vi "Build Address Tree.vi"(8 "error in (no error)":errorcluster, 10 "variant":variant, 11 "Addresses":refnum<vi>) -> (0 "error out":errorcluster, 2 "duplicate variant":variant)   [LabVIEW 2019, in "J1939 Workspace Shared.lvlib"]
uses:
  J1939 Workspace Shared.lvlib
  <vilib>/Utility/miscctls.llb/LVNodeAndColumnTypeDef.ctl
  <vilib>/picture/picture.llb/imagedata.ctl
  Addon/Addon Shared/Types/Address Lookup Table Data.ctl
  Addon/Addon Shared/J1939 Addon Shared.lvlib
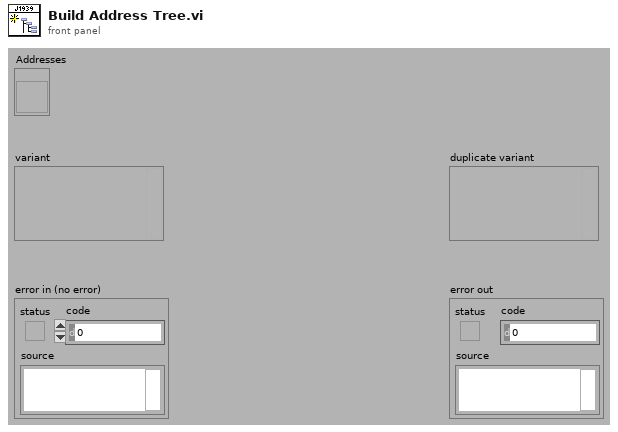
[diagram p1: front panel]
types:
  T1 = typedef "LVNodeAndColumnTypeDef.ctl" = cluster{"Node":string, "Column":i32}
  T2 = typedef "imagedata.ctl" = cluster{"image type":i32, "image depth":i32, "image":u8[], "mask":u8[], "colors":u32[], "Rectangle":cluster{"left":i16, "top":i16, "right":i16, "bottom":i16}}
  T3 = typedef "J1939 Addon Shared.lvlib/Address Lookup Table Data.ctl" = cluster{"Name":u8[], "Address":u8}
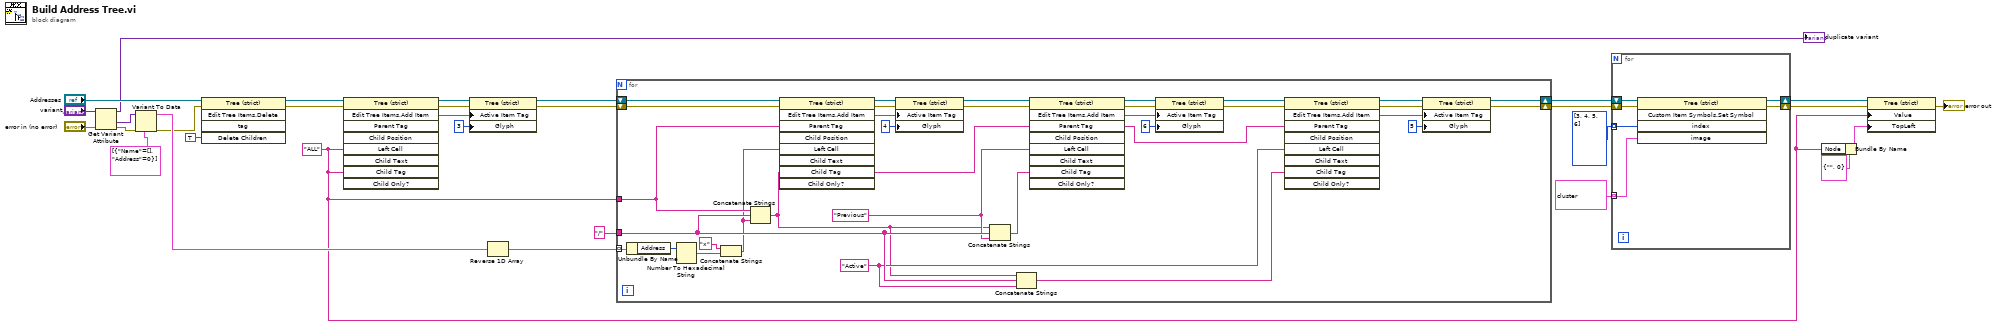
[diagram p0: block diagram]
diagram:
  w3 = "ALL" ("Left Cell String")
  n1 = Get Variant Attribute(Variant="variant", error in="error in (no error)") -> (duplicate Variant=→"duplicate variant":variant, values=w22:variant[], error out=w23:errorcluster)  [unwired: 2 in, 1 out]
  n2 = Variant To Data(error in=w23, type=T3[] [{"Name"=[], "Address"=0}], Variant=w22) -> (data=w21:T3[], error out=w18:errorcluster)
  n3 = invoke on="Invoke Node" class="Tree (strict)" method="Edit Tree Items.Delete"(reference="Addresses", error in=w18, "Delete Children"=TRUE ("Delete Children?")) -> (reference out=w29:refnum<vi>, error out=w28:errorcluster)  [unwired: 2 in, 3 out]
  n4 = invoke on="Invoke Node" class="Tree (strict)" method="Edit Tree Items.Add Item"(reference=w29, error in=w28, "Left Cell"=w3, "Child Tag"=w3) -> (reference out=w13:refnum<vi>, error out=w15:errorcluster, "Edit Tree Items:Add Item"=w16:string)  [unwired: 5 in, 6 out]
  n5 = property class="Tree (strict)"(reference=w13, error in=w15, "Active Item Tag"=w16, "Glyph"=3 ("Active Item:Symbol Index")) -> (reference out=w9:refnum<vi>, error out=w14:errorcluster)
  n6 = Reverse 1D Array(array=w21) -> (reversed array=w26:T3[])
  n7 = for {
    tunnel: w3 -> [w60]
    tunnel: w26 -> [w61] mode=indexing
    tunnel: "/" ("string") -> [w59]
    shift-right: [w37] -> w10
    shift-left: w14 -> [w62]
    shift-right: [w36] -> w8
    shift-left: w9 -> [w35]
    w56 = "Active" ("string")
    w55 = "Previous" ("string")
    n8 = Unbundle By Name(w61) -> ("Address"=w33:u8)
    n9 = Number To Hexadecimal String(2:w33) -> (0:w34:string)  [unwired: 1 in]
    n10 = Concatenate Strings("x" ("string"), w34) -> (w32:string)
    n11 = Concatenate Strings(w60, w59, w32) -> (w42:string)
    n12 = invoke on="Invoke Node" class="Tree (strict)" method="Edit Tree Items.Add Item"(reference=w35, error in=w62, "Parent Tag"=w60, "Left Cell"=w32, "Child Tag"=w42) -> (reference out=w53:refnum<vi>, error out=w52:errorcluster, "Edit Tree Items:Add Item"=w51:string)  [unwired: 4 in, 6 out]
    n13 = property class="Tree (strict)"(reference=w53, error in=w52, "Active Item Tag"=w51, "Glyph"=4 ("Active Item:Symbol Index")) -> (reference out=w50:refnum<vi>, error out=w49:errorcluster)
    n14 = Concatenate Strings(w42, w59, w55) -> (w58:string)
    n15 = Concatenate Strings(w42, w59, w56) -> (w57:string)
    n16 = invoke on="Invoke Node" class="Tree (strict)" method="Edit Tree Items.Add Item"(reference=w50, error in=w49, "Parent Tag"=w42, "Left Cell"=w55, "Child Tag"=w58) -> (reference out=w47:refnum<vi>, error out=w46:errorcluster, "Edit Tree Items:Add Item"=w45:string)  [unwired: 4 in, 6 out]
    n17 = property class="Tree (strict)"(reference=w47, error in=w46, "Active Item Tag"=w45, "Glyph"=6 ("Active Item:Symbol Index")) -> (reference out=w43:refnum<vi>, error out=w44:errorcluster)
    n18 = invoke on="Invoke Node" class="Tree (strict)" method="Edit Tree Items.Add Item"(reference=w43, error in=w44, "Parent Tag"=w42, "Left Cell"=w56, "Child Tag"=w57) -> (reference out=w40:refnum<vi>, error out=w38:errorcluster, "Edit Tree Items:Add Item"=w39:string)  [unwired: 4 in, 6 out]
    n19 = property class="Tree (strict)"(reference=w40, error in=w38, "Active Item Tag"=w39, "Glyph"=5 ("Active Item:Symbol Index")) -> (reference out=w36:refnum<vi>, error out=w37:errorcluster)
  }
  n20 = for {
    shift-right: [w67] -> w6
    shift-left: w10 -> [w65]
    tunnel: i32[] [3, 4, 5, 6] -> [w66] mode=indexing
    tunnel: T2[] [{"image type"=0, "image depth"=32, "image"=array[1024 elements], "mask"=[3, 192, 7, 224, 3, 224, 3, 224, 3, 224, 3, 192, 3, 192, 3, 192, 248, 191, 248, 159, 249, 159, 255, 255, 248, 30, 248, 30, 120, 30, 0, 0], "colors"=[], "Rectangle"={"left"=0, "top"=0, "right"=16, "bottom"=16}}, {"image type"=0, "image depth"=32, "image"=array[1024 elements], "mask"=[0, 0, 0, 0, 3, 128, 15, 224, 63, 248, 255, 254, 255, 255, 255, 255, 255, 255, 255, 255, 127, 255, 63, 255, 15, 255, 3, 255, 0, 254, 0, 0], "colors"=[], "Rectangle"={"left"=0, "top"=0, "right"=16, "bottom"=16}}, {"image type"=0, "image depth"=32, "image"=[0, 0, 0, 0, 0, 0, 0, 0, 0, 0, 0, 0, 0, 0, 0, 0, 2, 64, 64, 64, 5, 64, 64, 64, 52, 100, 18, 18, 115, 111, 10, 10, 94, 102, 17, 17, 62, 94, 26, 26, 16, 64, 64, 64, 10, 64, 64, 64, 5, 64, 64, 64, 2, 64, 64, 64, 0, 0, 0, 0, 0, 0, 0, 0, 0, 0, 0, 0, 0, 0, 0, 0, 2, 64, 64, 64, 5, 64, 64, 64, 132, 117, 12, 12, 247, 130, 6, 6, 255, 128, 0, 0, 255, 146, 35, 34, 255, 155, 52, 51, 255, 128, 0, 0, 241, 129, 13, 13, 144, 109, 19, 19, 28, 64, 64, 64, 14, 64, 64, 64, 4, 64, 64, 64, 1, 64, 64, 64, 0, 0, 0, 0, 2, 64, 64, 64, 36, 114, 12, 12, 220, 127, 12, 12, 255, 137, 16, 16, 255, 215, 134, 129, 255, 244, 173, 166, 255, 246, 174, 166, 255, 246, 174, 166, 255, 244, 173, 166, 255, 227, 153, 147, 255, 137, 16, 15, 227, 122, 14, 14, 41, 64, 63, 63, 19, 64, 64, 64, 6, 64, 64, 64, 0, 0, 0, 0, 5, 64, 64, 64, 220, 127, 11, 11, 255, 159, 45, 42, 255, 240, 145, 136, 255, 248, 147, 137, 255, 249, 147, 137, 255, 237, 164, 156, 255, 238, 170, 163, 255, 243, 147, 137, 255, 247, 147, 137, 255, 239, 145, 136, 255, 158, 44, 41, 231, 120, 14, 14, 46, 64, 64, 64, 21, 64, 64, 64, 2, 64, 64, 64, 132, 116, 11, 11, 255, 136, 11, 10, 255, 236, 118, 106, 255, 249, 121, 108, 255, 254, 126, 113, 255, 248, 127, 114, 255, 255, 255, 255, 255, 255, 255, 255, 255, 239, 137, 126, 255, 254, 126, 112, 255, 248, 121, 108, 255, 235, 118, 106, 255, 135, 10, 10, 178, 98, 29, 29, 51, 64, 64, 64, 5, 64, 64, 64, 247, 129, 3, 3, 255, 204, 71, 60, 255, 244, 95, 80, 255, 254, 102, 86, 255, 255, 110, 95, 255, 248, 111, 96, 255, 255, 255, 255, 255, 255, 255, 255, 255, 239, 123, 110, 255, 255, 110, 94, 255, 254, 102, 86, 255, 243, 95, 80, 255, 202, 71, 60, 251, 125, 5, 4, 107, 64, 64, 64, 52, 99, 17, 17, 255, 128, 0, 0, 255, 230, 71, 54, 255, 250, 76, 58, 255, 255, 88, 69, 255, 255, 94, 77, 255, 248, 94, 78, 255, 255, 255, 255, 255, 255, 255, 255, 255, 239, 109, 95, 255, 255, 94, 77, 255, 255, 87, 69, 255, 249, 76, 58, 255, 228, 71, 54, 255, 128, 0, 0, 171, 75, 50, 50, 115, 110, 9, 9, 255, 140, 10, 7, 255, 232, 55, 37, 255, 252, 62, 42, 255, 255, 75, 55, 255, 255, 81, 63, 255, 248, 80, 63, 255, 255, 255, 255, 255, 255, 255, 255, 255, 239, 97, 83, 255, 255, 81, 63, 255, 255, 74, 54, 255, 252, 61, 42, 255, 231, 54, 36, 255, 139, 9, 7, 205, 90, 36, 36, 94, 100, 15, 15, 255, 145, 13, 9, 255, 232, 49, 31, 255, 252, 57, 36, 255, 255, 70, 50, 255, 255, 76, 58, 255, 248, 76, 58, 255, 255, 255, 255, 255, 255, 255, 255, 255, 239, 93, 79, 255, 255, 76, 57, 255, 255, 69, 49, 255, 252, 56, 36, 255, 230, 49, 31, 255, 143, 12, 9, 200, 81, 44, 44, 62, 93, 26, 26, 255, 128, 0, 0, 255, 226, 48, 30, 255, 249, 54, 34, 255, 255, 67, 47, 255, 255, 75, 56, 255, 248, 75, 57, 255, 255, 255, 255, 255, 255, 255, 255, 255, 239, 92, 76, 255, 255, 75, 55, 255, 255, 66, 46, 255, 248, 54, 34, 255, 225, 48, 30, 255, 128, 0, 0, 190, 73, 52, 52, 16, 64, 64, 64, 241, 126, 6, 6, 255, 205, 41, 26, 255, 241, 51, 32, 255, 254, 60, 40, 255, 255, 71, 50, 255, 247, 73, 54, 255, 230, 138, 128, 255, 232, 153, 145, 255, 239, 80, 63, 255, 255, 70, 50, 255, 254, 59, 39, 255, 239, 51, 32, 255, 203, 40, 26, 249, 122, 9, 9, 172, 64, 64, 64, 10, 64, 64, 64, 144, 106, 19, 19, 255, 133, 4, 3, 255, 225, 48, 30, 255, 245, 53, 33, 255, 254, 60, 39, 255, 240, 93, 77, 255, 255, 255, 255, 255, 255, 255, 255, 255, 239, 137, 126, 255, 254, 59, 39, 255, 244, 52, 33, 255, 223, 48, 30, 255, 132, 4, 3, 207, 92, 35, 35, 152, 64, 64, 64, 5, 64, 64, 64, 28, 64, 64, 64, 227, 120, 10, 10, 255, 147, 13, 9, 255, 224, 48, 30, 255, 240, 51, 32, 255, 242, 53, 34, 255, 235, 126, 115, 255, 236, 133, 123, 255, 237, 59, 41, 255, 239, 51, 32, 255, 222, 48, 30, 255, 146, 13, 9, 241, 114, 15, 15, 146, 64, 64, 64, 106, 64, 64, 64, 2, 64, 64, 64, 14, 64, 64, 64, 66, 91, 36, 36, 231, 118, 11, 11, 255, 132, 4, 3, 255, 187, 34, 22, 255, 224, 48, 30, 255, 230, 49, 31, 255, 230, 49, 31, 255, 223, 48, 30, 255, 194, 38, 25, 255, 132, 4, 3, 241, 114, 15, 15, 147, 64, 64, 64, 109, 64, 64, 64, 51, 64, 64, 64, 0, 0, 0, 0, 5, 64, 64, 64, 21, 64, 64, 64, 51, 64, 64, 64, 179, 97, 29, 29, 251, 125, 4, 4, 255, 128, 0, 0, 255, 134, 8, 6, 255, 137, 11, 9, 255, 128, 0, 0, 249, 121, 9, 9, 207, 92, 35, 35, 146, 64, 64, 64, 109, 64, 64, 64, 47, 64, 64, 64, 21, 64, 64, 64, 0, 0, 0, 0, 2, 64, 64, 64, 7, 64, 64, 64, 23, 64, 64, 64, 53, 64, 64, 64, 107, 64, 64, 64, 171, 75, 50, 50, 205, 89, 35, 35, 200, 81, 44, 44, 190, 73, 52, 52, 172, 64, 64, 64, 152, 64, 64, 64, 106, 64, 64, 64, 51, 64, 64, 64, 21, 64, 64, 64, 6, 64, 64, 64], "mask"=[0, 0, 15, 240, 31, 248, 63, 252, 127, 254, 127, 254, 127, 255, 127, 255, 127, 255, 127, 255, 127, 255, 127, 255, 63, 254, 31, 252, 15, 248, 3, 240], "colors"=[], "Rectangle"={"left"=0, "top"=0, "right"=16, "bottom"=16}}, {"image type"=0, "image depth"=32, "image"=array[1024 elements], "mask"=[1, 128, 3, 192, 3, 192, 7, 224, 7, 224, 15, 240, 15, 240, 31, 248, 31, 248, 63, 252, 63, 252, 127, 254, 127, 254, 255, 255, 255, 255, 255, 255], "colors"=[], "Rectangle"={"left"=0, "top"=0, "right"=16, "bottom"=16}}] -> [w64] mode=indexing
    shift-right: [w63] -> w4
    shift-left: w8 -> [w68]
    n21 = invoke on="Invoke Node" class="Tree (strict)" method="Custom Item Symbols.Set Symbol"(reference=w68, error in=w65, "index"=w66, "image"=w64) -> (reference out=w63:refnum<vi>, error out=w67:errorcluster)  [unwired: 1 in, 3 out]
  }
  n22 = Bundle By Name(cluster=T1 {"Node"="", "Column"=0} ("Top Left Visible Cell"), "Node"=w3) -> (w1:T1)
  n23 = property class="Tree (strict)"(reference=w4, error in=w6, "Value"=w3, "TopLeft"=w1) -> (error out=→"error out":errorcluster)  [unwired: 1 out]
